vi "Bufor.vi"(10 "IN HI / IN LO 2":dynamicdata(graph), 11 "IN HI / IN LO":dynamicdata(graph)) -> (3 "Waveform Graph":dynamicdata(graph))   [LabVIEW 2021]
panel:
  out "Waveform":waveform(dbl)
  # "Realny sygnał wchodzący do przetwornika"
  # "Realny sygnał wchodzący do przetwornika"
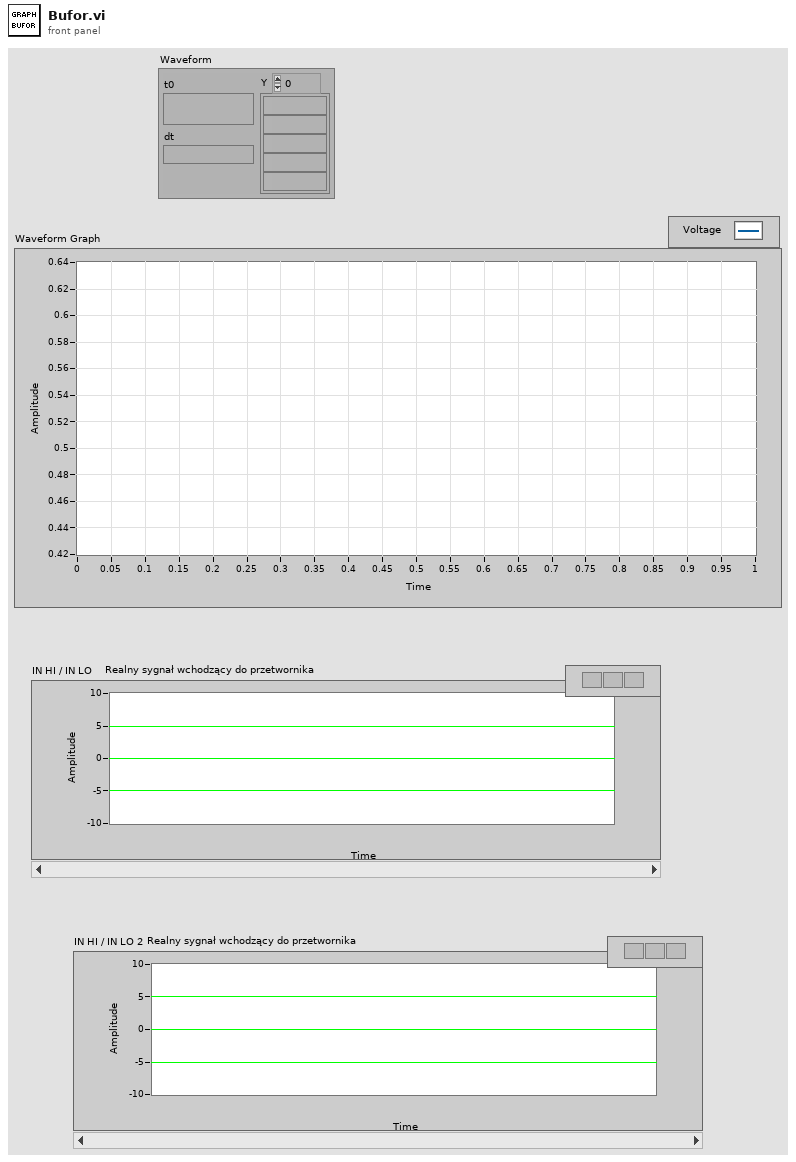
[diagram p1: front panel]
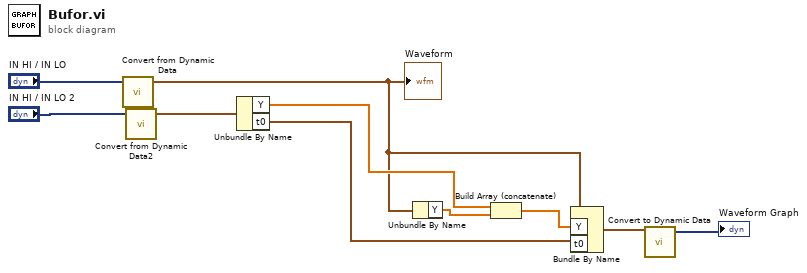
[diagram p0: block diagram]
diagram:
  n1 = call "Convert from Dynamic Data"("Dynamic Data Type"="IN HI / IN LO") -> ("Waveform"=w5:waveform(dbl))  [unwired: 3 in]
  "Waveform" <- w5
  n2 = call "Convert from Dynamic Data2"("Dynamic Data Type"="IN HI / IN LO 2") -> ("Waveform"=w10:waveform(dbl))  [unwired: 3 in]
  n3 = Unbundle By Name(w10) -> ("Y"=w8:dbl[], "t0"=w9:timestamp)
  n4 = Unbundle By Name(w5) -> ("Y"=w7:dbl[])
  n5 = Build Array (concatenate)(w8, w7) -> (w6:dbl[])
  n6 = Bundle By Name(cluster=w5, "Y"=w6, "t0"=w9) -> (w2:waveform(dbl))
  n7 = call "Convert to Dynamic Data"("Waveform"=w2) -> ("Dynamic Data Type"=→"Waveform Graph":dynamicdata)  [unwired: 3 in]
